vi "公式复合写入.vi"(11 "公式":cluster{"X^2":dbl, "X":dbl, "b":dbl}) -> ()   [LabVIEW 2016, in "斯坦道CODMn新电路板.lvlib"]
uses:
  <vilib>/Utility/miscctls.llb/LVPointTypeDef.ctl
panel:
  out "连接的字符串":string
  in  "参数下拉列表":enum16{"CODMn"}(ring)
  in  "量程下拉列表":enum16{"低量程1", "低量程2", "高量程1", "高量程2"}(ring)
  in  "取消":bool
  in  "确认":bool
  in  "加标回收":bool
  in  "标样核查":bool
  in  "跨度核查":bool
  in  "空白核查":bool
  in  "水样测量":bool=TRUE
  # "请选择要写入的参数"
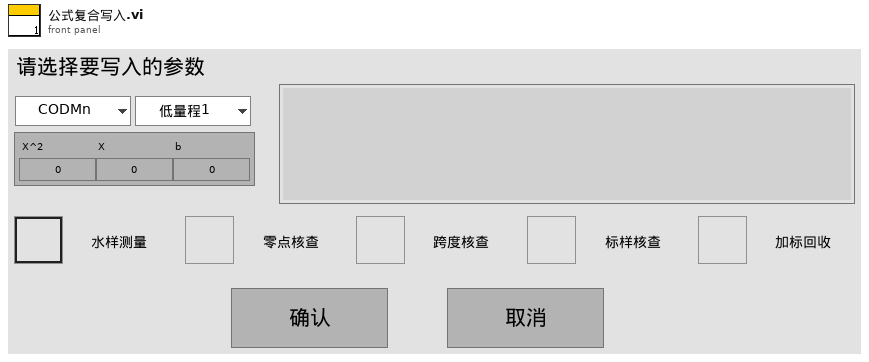
[diagram p1: front panel]
types:
  T1 = typedef "LVPointTypeDef.ctl" = cluster{"Horizontal":i16, "Vertical":i16}
  T2 = enum16{"", "水样测量", "标样核查", "零点核查", "跨度核查", "空白测试", "平行样测试", "加标回收"}
  T3 = cluster{"测量量程":dbl, "测量精度":dbl, "测量间隔":dbl, "消解温度":dbl, "消解时长":dbl, "空白校准时间":timestamp, "曲线截距":dbl, "曲线斜率":dbl, "测量检出限":dbl, "测量信号值":dbl, "线性相关系数":dbl, "二次多项式系数":dbl, "标样校准时间":timestamp, "稀释倍数":dbl, "三项式系数":dbl, "空白标定系数":dbl, "量程系数":dbl, "F0/ORPA":dbl, "F1/ORPB":dbl, "F2/ORPK":dbl, "F3":dbl, "F4":dbl, "F5":dbl, "F6":dbl, "F7":dbl, "X0/滴定数":dbl, "量程":dbl}
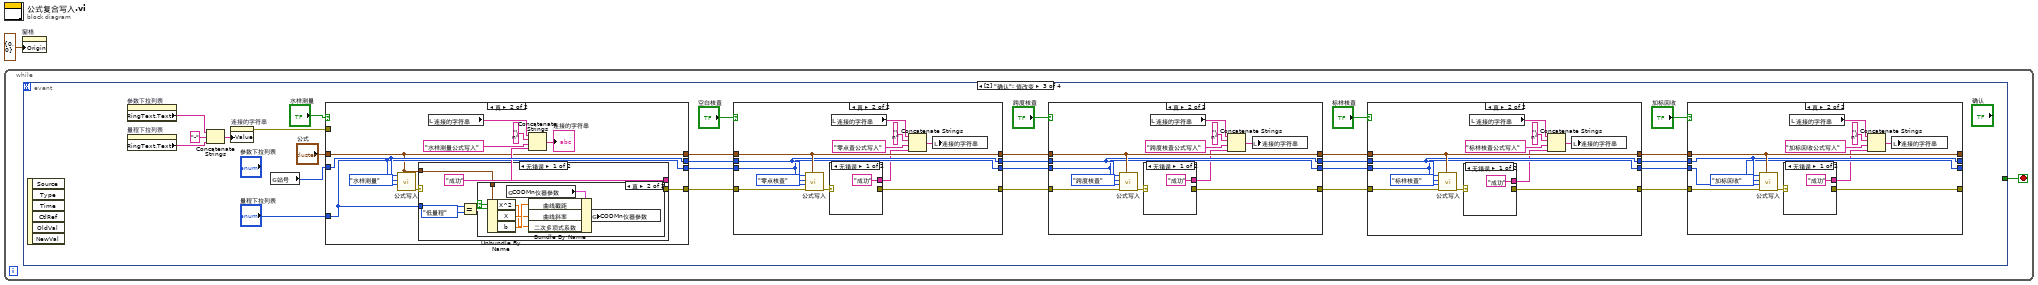
[diagram p0: block diagram]
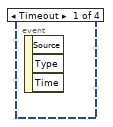
[diagram p2: hidden frame]
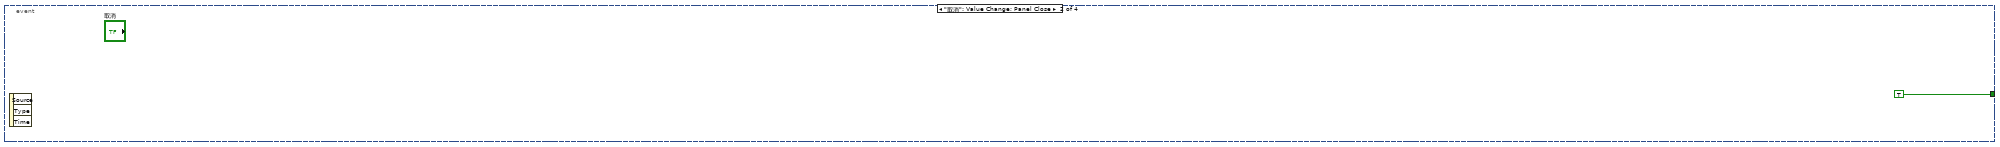
[diagram p3: hidden frame]
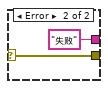
[diagram p5: hidden frame]
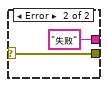
[diagram p7: hidden frame]
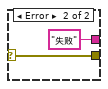
[diagram p9: hidden frame]
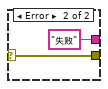
[diagram p11: hidden frame]
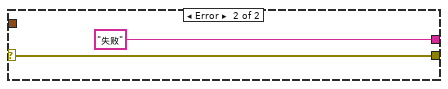
[diagram p14: hidden frame]
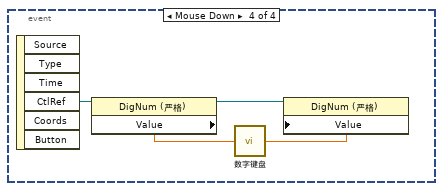
[diagram p15: hidden frame]
diagram:
  n1 = while {
    stop <- w2 stop-if-true
    n2 = event shown="[2] \"确认\": 值改变" {
      selector: _ -> [_ _ _ _]
      dyn-events: _ -> [_ _ _ _]
      timeout: _ -> [_ _ _ _]
      tunnel: [_ TRUE _ _] -> w2
      event Timeout {
        n3 = event-data() -> ()  [unwired: 1 in, 3 out]
      }
      event "取消": Value Change; Panel Close {
        n4 = event-data() -> ()  [unwired: 1 in, 3 out]
      }
      event "确认": Value Change {
        n5 = event-data() -> ()  [unwired: 1 in, 6 out]
        n6 = property on="参数下拉列表" class="Enum (严格)"() -> ("RingText.Text"=w7:string)  [unwired: 2 in, 2 out]
        n7 = property on="量程下拉列表" class="Enum (严格)"() -> ("RingText.Text"=w6:string)  [unwired: 2 in, 2 out]
        n8 = Concatenate Strings(w7, "-" ("字符串"), w6) -> (w8:string)
        n9 = property on="连接的字符串" class="Str"("Value"=w8) -> (error out=w9:errorcluster)  [unwired: 2 in, 1 out]
        n10 = global read "CODMn断电保存全局变量.vi" "站号"() -> (w4:u16)
        n11 = case shown="真" "水样测量" {
          tunnel: "公式" -> [w107 w109]
          tunnel: w4 -> [w106 w118]
          tunnel: "量程下拉列表" -> [w105 w110]
          tunnel: [w107 w109] -> w29
          tunnel: [w106 w118] -> w28
          tunnel: [w105 w110] -> w27
          tunnel: [_ w116] -> w11
          tunnel: w9 -> [_ _]
          frame False {
          }
          frame True {
            n12 = call "公式写入.vi"("公式"=w109, "量程"=w110, "测量模式"=T2."水样测量", "测量参数"=w118) -> ("error out"=w117:errorcluster)  [unwired: 7 in]
            n13 = case shown="无错误" w117 {
              selector: w117 -> [_ w131]
              tunnel: [_ w131] -> w116
              tunnel: ["成功" "失败"] -> w115
              tunnel: w110 -> [w122 _]
              tunnel: w109 -> [w119 _]
              frame No Error {
                n14 = Equal?(x=w122, y=enum16{"低量程", "高量程"}."低量程") -> (x = y?=w120:bool)
                n15 = case shown="真" w120 {
                  tunnel: w119 -> [_ w124]
                  frame False {
                  }
                  frame True {
                    n16 = Unbundle By Name(w124) -> ("X^2"=w127:dbl, "X"=w128:dbl, "b"=w129:dbl)
                    n17 = global read "CODMn断电保存全局变量.vi" "CODMn仪器参数"() -> (w126:T3)
                    n18 = Bundle By Name(cluster=w126, "曲线截距"=w129, "曲线斜率"=w128, "二次多项式系数"=w127) -> (w125:T3)
                    n19 = global write "CODMn断电保存全局变量.vi" "CODMn仪器参数"(w125) -> ()
                  }
                }
              }
              frame Error {
              }
            }
            n20 = local read "连接的字符串"() -> (w112:string)
            n21 = Concatenate Strings(w112, "\n" ("字符串"), "水样测量公式写入", w115) -> (→"连接的字符串":string)
          }
        }
        n22 = case shown="真" "空白核查" {
          tunnel: w29 -> [w89 w101]
          tunnel: w28 -> [w88 w100]
          tunnel: w27 -> [w87 w99]
          tunnel: [_ w94] -> w26
          tunnel: [w89 w101] -> w25
          tunnel: [w88 w100] -> w24
          tunnel: [w87 w99] -> w23
          tunnel: w11 -> [_ w98]
          frame False {
          }
          frame True {
            n23 = call "公式写入.vi"("公式"=w101, "error in (no error)"=w98, "量程"=w99, "测量模式"=T2."零点核查", "测量参数"=w100) -> ("error out"=w95:errorcluster)  [unwired: 6 in]
            n24 = case shown="无错误" w95 {
              selector: w95 -> [_ w104]
              tunnel: [_ w104] -> w94
              tunnel: ["成功" "失败"] -> w96
              frame No Error {
              }
              frame Error {
              }
            }
            n25 = local read "连接的字符串"() -> (w93:string)
            n26 = Concatenate Strings(w93, "\n" ("字符串"), "零点查公式写入", w96) -> (w91:string)
            n27 = local write "连接的字符串"(w91) -> ()
          }
        }
        n28 = case shown="真" "跨度核查" {
          tunnel: w25 -> [w71 w83]
          tunnel: w24 -> [w70 w82]
          tunnel: w23 -> [w69 w81]
          tunnel: [w71 w83] -> w22
          tunnel: [w70 w82] -> w20
          tunnel: [w69 w81] -> w19
          tunnel: w26 -> [_ w80]
          tunnel: [_ w73] -> w10
          frame False {
          }
          frame True {
            n29 = call "公式写入.vi"("公式"=w83, "error in (no error)"=w80, "量程"=w81, "测量模式"=T2."跨度核查", "测量参数"=w82) -> ("error out"=w74:errorcluster)  [unwired: 6 in]
            n30 = case shown="无错误" w74 {
              selector: w74 -> [_ w86]
              tunnel: [_ w86] -> w73
              tunnel: ["成功" "失败"] -> w75
              frame No Error {
              }
              frame Error {
              }
            }
            n31 = local read "连接的字符串"() -> (w77:string)
            n32 = Concatenate Strings(w77, "\n" ("字符串"), "跨度核查公式写入", w75) -> (w79:string)
            n33 = local write "连接的字符串"(w79) -> ()
          }
        }
        n34 = case shown="真" "标样核查" {
          tunnel: w22 -> [w53 w65]
          tunnel: w20 -> [w52 w64]
          tunnel: w19 -> [w51 w63]
          tunnel: [_ w55] -> w16
          tunnel: [w53 w65] -> w21
          tunnel: [w52 w64] -> w18
          tunnel: [w51 w63] -> w17
          tunnel: w10 -> [_ w62]
          frame False {
          }
          frame True {
            n35 = call "公式写入.vi"("公式"=w65, "error in (no error)"=w62, "量程"=w63, "测量模式"=T2."标样核查", "测量参数"=w64) -> ("error out"=w56:errorcluster)  [unwired: 6 in]
            n36 = case shown="无错误" w56 {
              selector: w56 -> [_ w68]
              tunnel: [_ w68] -> w55
              tunnel: ["成功" "失败"] -> w57
              frame No Error {
              }
              frame Error {
              }
            }
            n37 = local read "连接的字符串"() -> (w59:string)
            n38 = Concatenate Strings(w59, "\n" ("字符串"), "标样核查公式写入", w57) -> (w61:string)
            n39 = local write "连接的字符串"(w61) -> ()
          }
        }
        n40 = case shown="真" "加标回收" {
          tunnel: w21 -> [w35 w47]
          tunnel: w18 -> [w34 w46]
          tunnel: w17 -> [w33 w45]
          tunnel: [w35 w47] -> _
          tunnel: [w34 w46] -> _
          tunnel: [w33 w45] -> _
          tunnel: w16 -> [_ w44]
          tunnel: [_ w37] -> _
          frame False {
          }
          frame True {
            n41 = call "公式写入.vi"("公式"=w47, "error in (no error)"=w44, "量程"=w45, "测量模式"=T2."加标回收", "测量参数"=w46) -> ("error out"=w38:errorcluster)  [unwired: 6 in]
            n42 = case shown="无错误" w38 {
              selector: w38 -> [_ w50]
              tunnel: [_ w50] -> w37
              tunnel: ["成功" "失败"] -> w39
              frame No Error {
              }
              frame Error {
              }
            }
            n43 = local read "连接的字符串"() -> (w41:string)
            n44 = Concatenate Strings(w41, "\n" ("字符串"), "加标回收公式写入", w39) -> (w43:string)
            n45 = local write "连接的字符串"(w43) -> ()
          }
        }
      }
      event "公式.X^2", "公式.X", "公式.b": Mouse Down {
        n46 = event-data() -> ("CtlRef"=w135:refnum<vi>)  [unwired: 1 in, 5 out]
        n47 = property class="DigNum (严格)"(reference=w135) -> (reference out=w132:refnum<vi>, "Value"=w134:dbl)  [unwired: 1 in, 1 out]
        n48 = call "数字键盘.vi"("OldNumber"=w134) -> ("NewNumber"=w133:dbl)
        n49 = property class="DigNum (严格)"(reference=w132, "Value"=w133) -> ()  [unwired: 1 in, 2 out]
      }
    }
  }
  n50 = property on="窗格" class="Pane"("Origin"=T1 {"Horizontal"=0, "Vertical"=0} ("原点")) -> ()  [unwired: 2 in, 2 out]
